vi "Same Name VI.vi"(11 "Numeric 2":dbl) -> (10 "Numeric 3":dbl)   [LabVIEW 2023]
panel:
  in  "Numeric":dbl
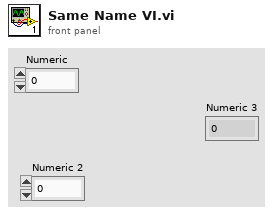
[diagram p1: front panel]
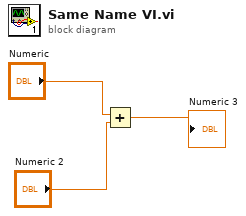
[diagram p0: block diagram]
diagram:
  n1 = Add(x="Numeric", y="Numeric 2") -> (x+y=→"Numeric 3":dbl)
